vi "ArrayToCluster.vi"(1 "N_r":i32, 2 "State Array":dbl[](array[numeric]), 3 "N_c":i32) -> (0 "State Cluster":T1)   [LabVIEW 2019]
panel:
  in  "Input State 2":T1
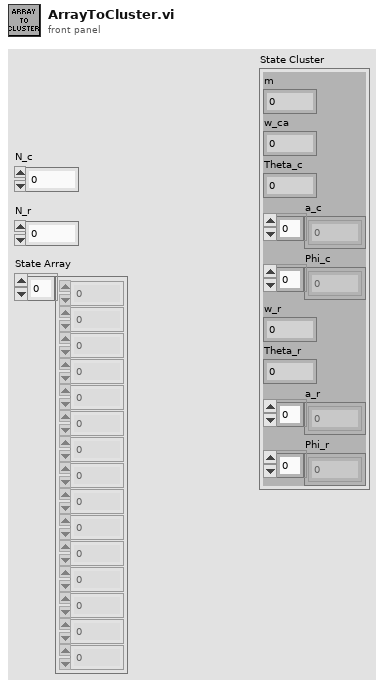
[diagram p1: front panel]
types:
  T1 = cluster{"m":dbl, "w_ca":dbl, "Theta_c":dbl, "a_c":dbl[], "Phi_c":dbl[], "w_r":dbl, "Theta_r":dbl, "a_r":dbl[], "Phi_r":dbl[]}
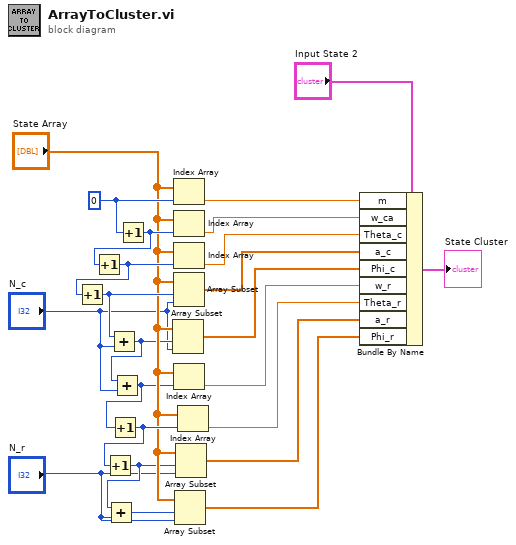
[diagram p0: block diagram]
diagram:
  w17 = 0 ("index")
  n1 = Increment(x=w17) -> (x+1=w16:i32)
  n2 = Increment(x=w16) -> (x+1=w15:i32)
  n3 = Increment(x=w15) -> (x+1=w14:i32)
  n4 = Add(x=w14, y="N_c") -> (x+y=w2:i32)
  n5 = Add(x=w2, y="N_c") -> (x+y=w3:i32)
  n6 = Increment(x=w3) -> (x+1=w11:i32)
  n7 = Increment(x=w11) -> (x+1=w8:i32)
  n8 = Add(x=w8, y="N_r") -> (x+y=w7:i32)
  n9 = Array Subset(array="State Array", index=w2, length="N_c") -> (w18:dbl[])
  n10 = Index Array(array="State Array", index=w17) -> (element=w22:dbl)
  n11 = Index Array(array="State Array", index=w16) -> (element=w21:dbl)
  n12 = Index Array(array="State Array", index=w15) -> (element=w20:dbl)
  n13 = Array Subset(array="State Array", index=w14, length="N_c") -> (w19:dbl[])
  n14 = Index Array(array="State Array", index=w3) -> (element=w13:dbl)
  n15 = Array Subset(array="State Array", index=w7, length="N_r") -> (w5:dbl[])
  n16 = Array Subset(array="State Array", index=w8, length="N_r") -> (w10:dbl[])
  n17 = Index Array(array="State Array", index=w11) -> (element=w12:dbl)
  n18 = Bundle By Name(cluster="Input State 2", "m"=w22, "w_ca"=w21, "Theta_c"=w20, "a_c"=w19, "Phi_c"=w18, "w_r"=w13, "Theta_r"=w12, "a_r"=w10, "Phi_r"=w5) -> (→"State Cluster":T1)
